vi "SimClimb.vi"() -> ()   [LabVIEW 2023]
uses:
  <vilib>/Rock Robotics/WPI/ThirdParty/JAS_Junk/TrajLib/Enum/DCMOTOR_TYPES_ENUM.ctl
  <vilib>/Rock Robotics/WPI/ThirdParty/JAS_Junk/TrajLib/VI/Util_GetTime_U32.vi
  <vilib>/Rock Robotics/WPI/ThirdParty/JAS_Junk/TrajLib/VI/numCmd_ObtainQueue_OneDbl.vi
  <vilib>/Rock Robotics/WPI/ThirdParty/JAS_Junk/TrajLib/SlewRateLimiter_New.vi
  <vilib>/Rock Robotics/WPI/ThirdParty/JAS_Junk/TrajLib/SlewRateLimiter_Reset.vi
  <vilib>/Rock Robotics/WPI/ThirdParty/JAS_Junk/TrajLib/SlewRateLimiter_Calculate.vi
  <vilib>/Rock Robotics/WPI/ThirdParty/JAS_Junk/TrajLib/SlewRateLimiter_SetRate.vi
  <vilib>/Rock Robotics/WPI/ThirdParty/JAS_Junk/TrajLib/VI/Util_GetTime_U64.vi
  <vilib>/Rock Robotics/WPI/ThirdParty/JAS_Junk/TrajLib/Trajectory_Library.lvlib
panel:
  out "R At Setpoint":bool
  out "R Rev / Lo Lim":bool
  out "R Fwd / Hi Lim":bool
  out "R Climb Control":T1(graph)
  out "Motor Current":dbl
  out "L Rev / Lo Lim":bool
  out "L Fwd / Hi Lim":bool
  out "L Climb Demand Inch":dbl
  out "Battery Voltage":dbl format="%10.1f"
  out "L Climb Control":T1(graph)
  out "L Pos Inch":dbl format="%13.1f"
  out "L AtSetpoint":bool
  in  "Claw Height Dmd Inches":dbl min=-1.0 max=23.0 step=1.0
  out "L Motor Dmd (CO)":dbl format="%10.3f"
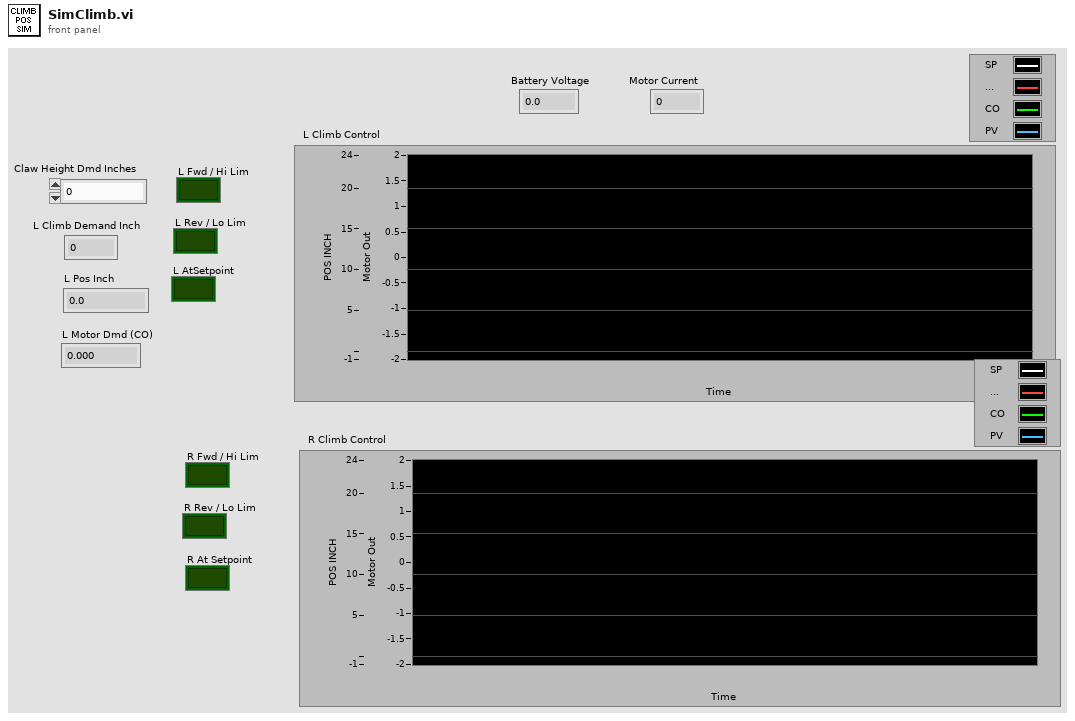
[diagram p1: front panel]
types:
  T1 = cluster{"Setpoint":dbl, "FeedForward":dbl, "CO-ControlOutput":dbl, "Velocity_RPM":dbl}
  T2 = typedef "Trajectory_Library.lvlib/DCMOTOR_TYPES_ENUM.ctl" = enum16{"CIM", "AndyMark 9015", "Andy Mark RS 775 125", "Bag", "BaneBots RS 550", "BaneBots RS 775", "Falcon 500", "Mini CIM", "NEO", "NEO 550", "Romi BuiltIn", "Vex 775 Pro", "Snow Blower AM 2235A", "Bosch Seat AM 3493"}
  T3 = typedef "Trajectory_Library.lvlib/LINEAR_SYSTEM_ID_ELEVATOR_MODEL.CTL" = cluster{"DCMOTOR_TYPES":T2, "Num Motors":i32, "WinchRadias_Meters":dbl, "mass_Kg":dbl, "Gearing":dbl}
  T4 = typedef "Trajectory_Library.lvlib/ELEVATOR_SIM_SIMULATION_PARAMS.ctl" = cluster{"MinHeight_Meters":dbl, "MaxHeight_Meters":dbl, "Measurment StdDev":dbl, "SimulateGravity":bool}
  T5 = cluster{"Claw Height Dmd Inches":dbl, "Left Dmd":dbl, "Left Output":dbl, dbl}
  T6 = cluster{"Claw Height Dmd Inches":dbl, "Right Demand":dbl, "Right Output":dbl, dbl}
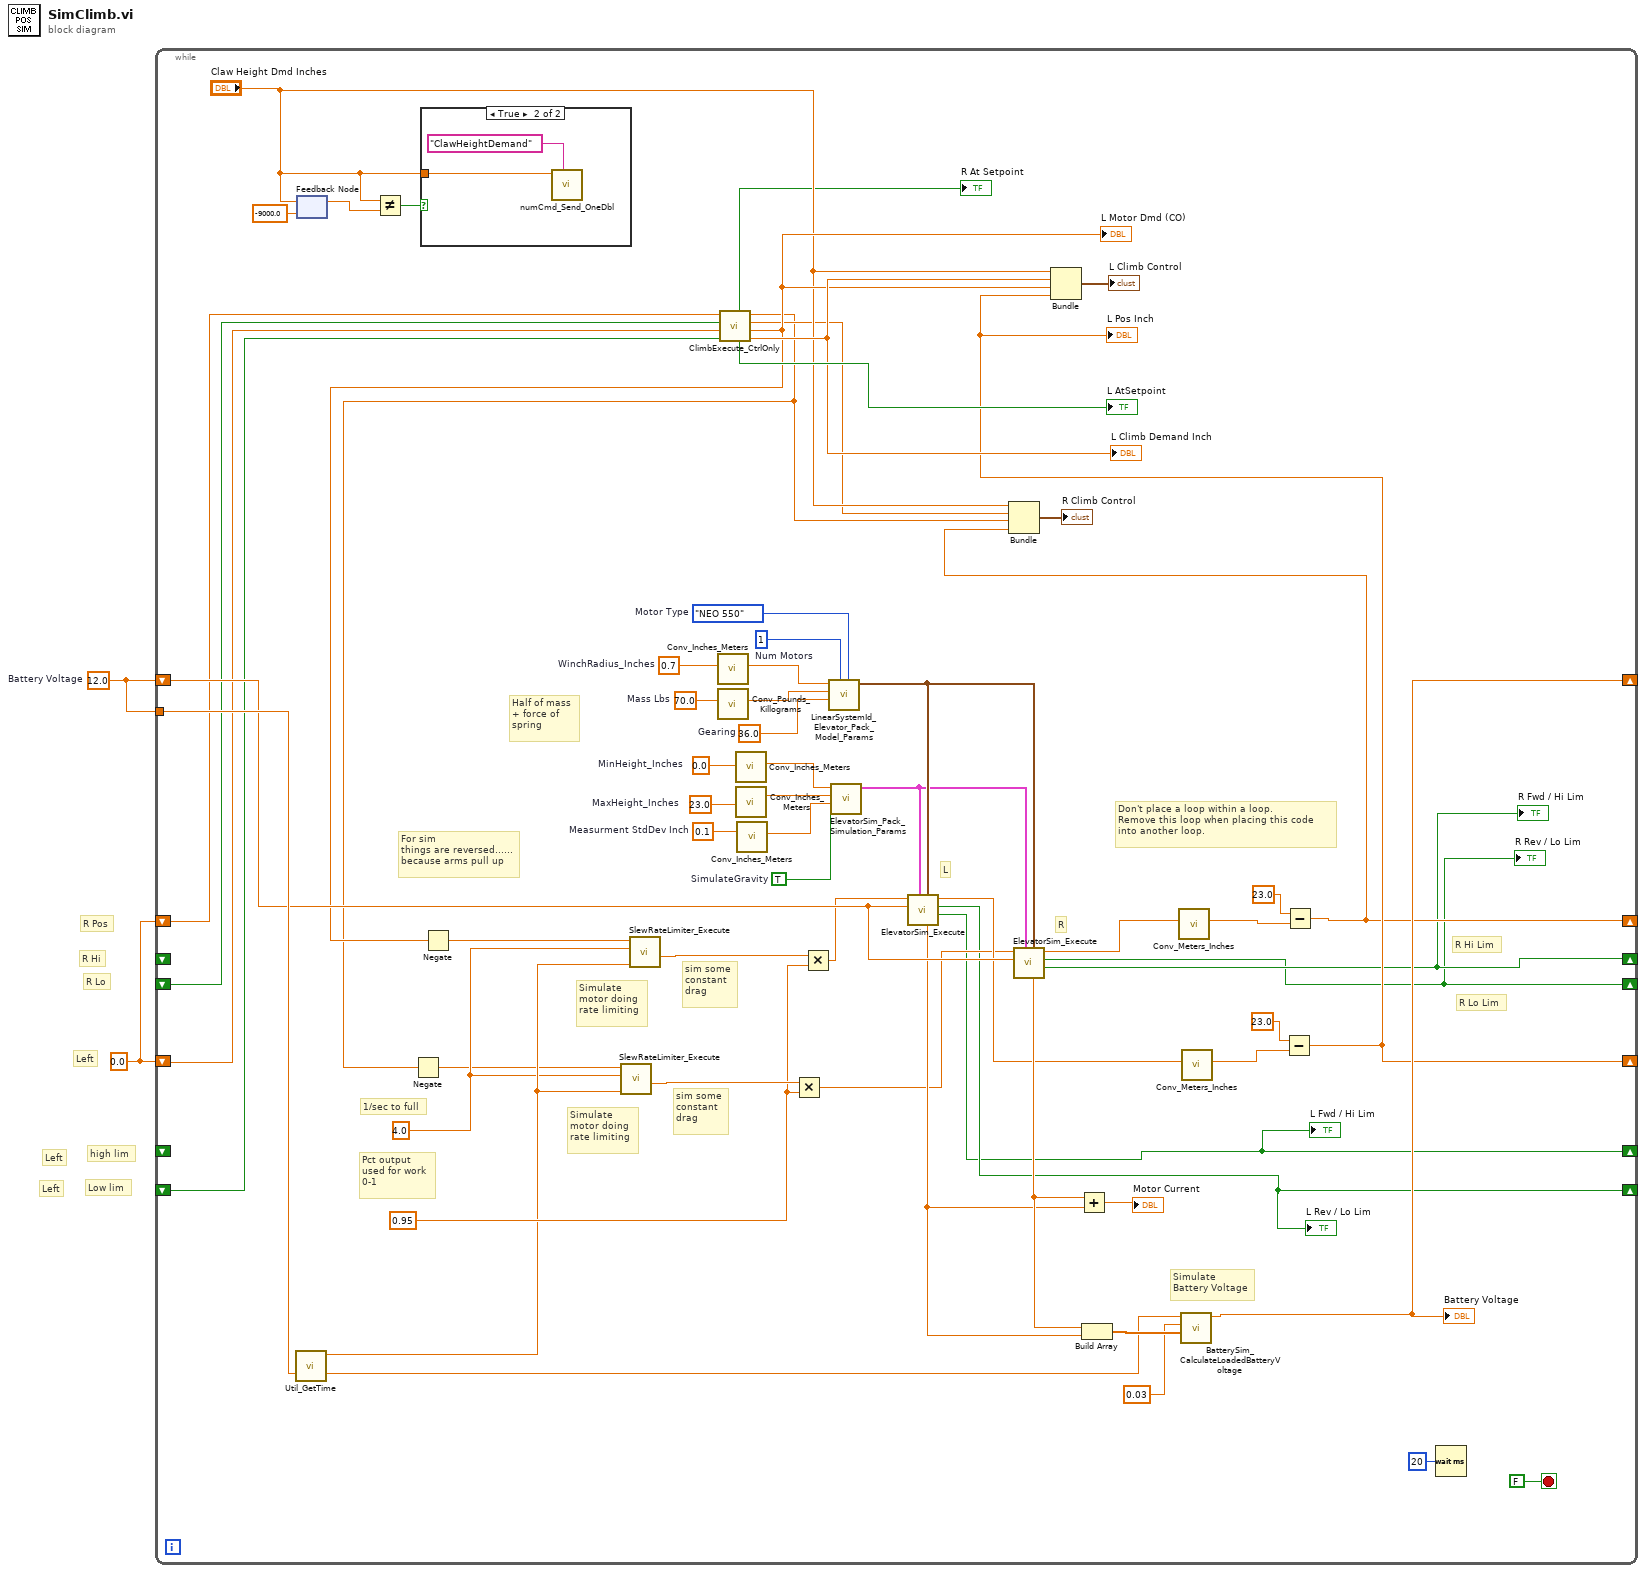
[diagram p0: block diagram]
diagram:
  w1 = 0.0 ("Degrees")
  w2 = 12.0  # Battery Voltage
  # "R Pos"
  # "R Lo"
  # "R Hi"
  # "Left"
  # "Left"
  # "Left"
  # "Low lim"
  # "high lim"
  n1 = while {
    shift-right: [w42] -> _
    shift-left: w2 -> [w39]
    shift-right: [w13] -> _
    shift-left: w1 -> [w29]
    tunnel: w2 -> [w41]
    shift-right: [w11] -> _
    shift-left: _ -> [_]
    shift-right: [w12] -> _
    shift-left: _ -> [w28]
    shift-right: [w6] -> _
    shift-left: w1 -> [w31]
    shift-right: [w4] -> _
    shift-left: _ -> [_]
    shift-right: [w3] -> _
    shift-left: _ -> [w30]
    stop <- FALSE stop-if-true
    w47 = 0.0  # MinHeight_Inches
    w48 = 23.0  # MaxHeight_Inches
    w49 = 0.1  # Measurment StdDev Inch
    w55 = TRUE  # SimulateGravity
    w53 = 0.7  # WinchRadius_Inches
    w56 = 36.0  # Gearing
    w51 = 70.0  # Mass Lbs
    w57 = 1  # Num Motors
    w58 = DCMOTOR_TYPES_ENUM."NEO 550"  # Motor Type
    w22 = 4.0 ("y")
    w24 = 0.95 ("y")
    # "For sim\nthings are reversed......\nbecause arms pull up"
    # "Simulate\nmotor doing\nrate limiting"
    # "sim some\nconstant\ndrag"
    # "R Lo Lim"
    # "R Hi Lim"
    # "R"
    # "L"
    # "Half of mass\n+ force of \nspring"
    # "Don't place a loop within a loop. \nRemove this loop when placing this code\ninto another loop."
    # "1/sec to full"
    # "Simulate\nBattery Voltage"
    # "Pct output\nused for work\n0-1"
    # "Simulate\nmotor doing\nrate limiting"
    # "sim some\nconstant\ndrag"
    n2 = call <vilib>:"Util_GetTime.vi"() -> ("FPGA_Time_Seconds"=w23:dbl)  [unwired: 9 in, 2 out]
    n3 = feedback-in #1("Claw Height Dmd Inches") -> ()
    n4 = feedback #1(-9000.0 ("Pos Dmd DEG")) -> (w60:dbl)
    n5 = Not Equal?(x="Claw Height Dmd Inches", y=w60) -> (x != y?=w61:bool)
    n6 = case shown="True" w61 {
      tunnel: "Claw Height Dmd Inches" -> [_ w66]
      frame False {
      }
      frame True {
        n7 = call <vilib>:"numCmd_Send_OneDbl.vi"("Command Name"="ClawHeightDemand", "Value"=w66) -> ()  [unwired: 9 in, 1 out]
      }
    }
    n8 = call <vilib>:"Conv_Inches_Meters.vi"("INCH"=w53) -> ("Meters"=w52:dbl)  [unwired: 10 in]
    n9 = call <vilib>:"Conv_Pounds_Killograms.vi"("Pounds"=w51) -> ("Killograms"=w50:dbl)  [unwired: 10 in]
    n10 = call "ClimbExecute_CtrlOnly.vi"("Left Hard Limit Rev"=w28, "Left Sensor Position"=w29, "Right Hard Limit Rev"=w30, "Right Sensor Position"=w31) -> ("Left Dmd"=w33:dbl, "Left Output"=w19:dbl, "Right Demand"=w8:dbl, "Right Output"=w7:dbl, "Left OnTarget"=→"L AtSetpoint":bool, "Right OnTarget"=→"R At Setpoint":bool)  [unwired: 2 in]
    "L Motor Dmd (CO)" <- w19
    "L Climb Demand Inch" <- w33
    n11 = Negate(x=w7) -> (-x=w18:dbl)
    n12 = Negate(x=w19) -> (-x=w20:dbl)
    n13 = call <vilib>:"SlewRateLimiter_Execute.vi"("Time"=w23, "PositiveRate"=w22, "Input"=w18) -> ("Output"=w26:dbl)  [unwired: 7 in, 1 out]
    n14 = call <vilib>:"SlewRateLimiter_Execute.vi"("Time"=w23, "PositiveRate"=w22, "Input"=w20) -> ("Output"=w62:dbl)  [unwired: 7 in, 1 out]
    n15 = call <vilib>:"Conv_Inches_Meters.vi"("INCH"=w47) -> ("Meters"=w46:dbl)  [unwired: 10 in]
    n16 = call <vilib>:"Conv_Inches_Meters.vi"("INCH"=w48) -> ("Meters"=w45:dbl)  [unwired: 10 in]
    n17 = call <vilib>:"Conv_Inches_Meters.vi"("INCH"=w49) -> ("Meters"=w44:dbl)  [unwired: 10 in]
    n18 = Multiply(x=w26, y=w24) -> (x*y=w25:dbl)
    n19 = Multiply(x=w62, y=w24) -> (x*y=w27:dbl)
    n20 = call <vilib>:"LinearSystemId_Elevator_Pack_Model_Params.vi"("DCMOTOR_TYPES"=w58, "Num Motors"=w57, "Gearing"=w56, "mass_Kg"=w50, "WinchRadius_Meters"=w52) -> ("Elevator_Model _Params"=w54:T3)  [unwired: 6 in]
    n21 = call <vilib>:"ElevatorSim_Pack_Simulation_Params.vi"("SimulateGravity"=w55, "Measurment StdDev"=w44, "MaxHeight_Meters"=w45, "MinHeight_Meters"=w46) -> ("ElevatorSim_Simulation _Params"=w21:T4)  [unwired: 7 in]
    n22 = call <vilib>:"ElevatorSim_Execute.vi"("LinearSystemID_Elevator_Model _Params"=w54, "ElevatorSim_Simulation _Params"=w21, "Battery Volts"=w39, "Motor Dmd"=w27) -> ("AtLowLimit"=w11:bool, "At HIgh LImit"=w12:bool, "ElevatorHeight_Meters"=w35:dbl, "Motor Current"=w37:dbl)  [unwired: 2 in, 2 out]
    "L Fwd / Hi Lim" <- w11
    "L Rev / Lo Lim" <- w12
    n23 = call <vilib>:"ElevatorSim_Execute.vi"("LinearSystemID_Elevator_Model _Params"=w54, "ElevatorSim_Simulation _Params"=w21, "Battery Volts"=w39, "Motor Dmd"=w25) -> ("AtLowLimit"=w4:bool, "At HIgh LImit"=w3:bool, "ElevatorHeight_Meters"=w32:dbl, "Motor Current"=w38:dbl)  [unwired: 2 in, 2 out]
    "R Fwd / Hi Lim" <- w4
    "R Rev / Lo Lim" <- w3
    n24 = Add(x=w38, y=w37) -> (x+y=→"Motor Current":dbl)
    n25 = Build Array(w38, w37) -> (w43:dbl[])
    n26 = call <vilib>:"Conv_Meters_Inches.vi"("Meters"=w32) -> ("Inches"=w16:dbl)  [unwired: 10 in]
    n27 = call <vilib>:"BatterySim_CalculateLoadedBatteryVoltage.vi"("Currents"=w43, "Resistance_Ohms"=0.03, "NominalVoltage"=w41) -> ("Voltage"=w42:dbl)  [unwired: 8 in]
    "Battery Voltage" <- w42
    n28 = call <vilib>:"Conv_Meters_Inches.vi"("Meters"=w35) -> ("Inches"=w14:dbl)  [unwired: 10 in]
    n29 = Subtract(x=23.0, y=w14) -> (x-y=w13:dbl)
    "L Pos Inch" <- w13
    n30 = Bundle("Claw Height Dmd Inches"="Claw Height Dmd Inches", "Left Dmd"=w33, "Left Output"=w19, w13) -> (→"L Climb Control":T5)  [unwired: 1 in]
    n31 = Subtract(x=23.0, y=w16) -> (x-y=w6:dbl)
    n32 = Bundle("Claw Height Dmd Inches"="Claw Height Dmd Inches", "Right Demand"=w8, "Right Output"=w7, w6) -> (→"R Climb Control":T6)  [unwired: 1 in]
    n33 = Wait (ms)(milliseconds to wait=u32 20) -> ()  [unwired: 1 out]
  }
